vi "Opdracht_1_StapGrootte.vi"(8 "fs":sgl, 11 "N":sgl) -> (1 "Stapgrootte":sgl, 2 "?":sgl)   [LabVIEW 2018]
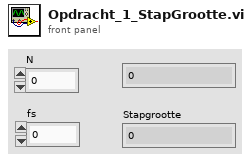
[diagram p1: front panel]
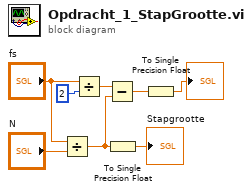
[diagram p0: block diagram]
diagram:
  n1 = Divide(x="fs", y="N") -> (x/y=w3:sgl)
  n2 = Divide(x="fs", y=u32 2) -> (x/y=w7:sgl)
  n3 = Subtract(x=w7, y=w3) -> (x-y=w5:sgl)
  n4 = To Single Precision Float(number=w3) -> (single precision float=→"Stapgrootte":sgl)
  n5 = To Single Precision Float(number=w5) -> (single precision float=→"?":sgl)
